vi "ADC_clock_temp.vi"(6 "phase":u8, 7 "converter box version":i16=1 min=1 max=2, 10 "iterations per cycle":u8=4, 11 "counter in":u8) -> (3 "counter out":u8)   [LabVIEW 2010]
uses:
  <vilib>/eio/EIONode/EIONode.xnode
  <vilib>/rvi/eio/nirviEIOImplementation/nirviEIOImplementation.xnode
  <vilib>/rvi/eio/common/nirviEmuClasses.ctl
  <vilib>/rvi/eio/common/nirviEmuTemplateMethod_noerrors.vi
panel:
  out "clock signal high?":bool
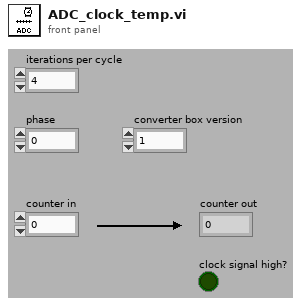
[diagram p1: front panel]
types:
  T1 = typedef "nirviEmuClasses.ctl" = enum16{"IO Read", "IO Write", "Method", "Property Read", "Property Write"}
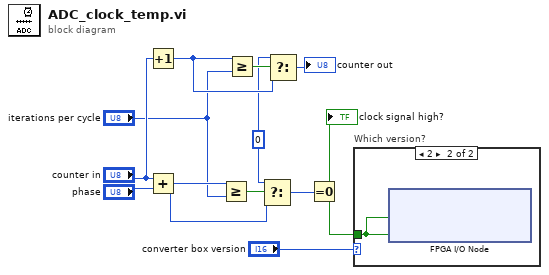
[diagram p0: block diagram]
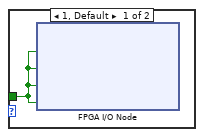
[diagram p2: hidden frame]
diagram:
  w1 = u8 0
  n1 = Increment(x="counter in") -> (x+1=w8:u8)
  n2 = Add(x="counter in", y="phase") -> (x+y=w5:u8)
  n3 = Greater Or Equal?(x=w5, y="iterations per cycle") -> (x >= y?=w6:bool)
  n4 = Greater Or Equal?(x=w8, y="iterations per cycle") -> (x >= y?=w11:bool)
  n5 = Select(t=w1, s=w6, f=w5) -> (s? t:f=w4:u8)
  n6 = Select(t=w1, s=w11, f=w8) -> (s? t:f=→"counter out":u8)
  n7 = Equal To 0?(x=w4) -> (x = 0?=w3:bool)
  "clock signal high?" <- w3
  n8 = case "Which version?" shown="2" "converter box version" {
    tunnel: w3 -> [w13 w58]
    frame 1, Default {
      n9 = xnode "FPGA I/O Node"("Connector2/DIO14"=w13, "Connector2/DIO15"=w13, "Connector1/DIO14"=w13, "Connector1/DIO15"=w13) -> ()  [unwired: 4 in, 4 out]
    }
    frame 2 {
      n10 = xnode "FPGA I/O Node"("Connector2/DIO15"=w58, "Connector1/DIO15"=w58) -> ()  [unwired: 2 in, 2 out]
    }
  }
